vi "NumericArrayResizeTest.vi"() -> ()   [LabVIEW 2010]
uses:
  new_bsvt_test/Debug/new_bsvt_test.dll
panel:
  out "initialized array":i8[](array[numeric])
  out "size(s)":i32
  out "return type":i8
  out "arg1":i8[](array[numeric])
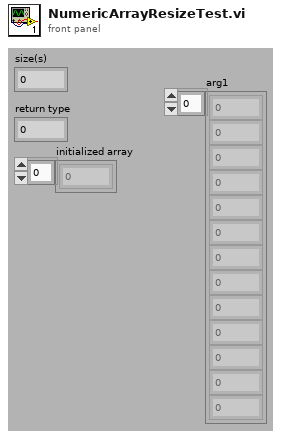
[diagram p1: front panel]
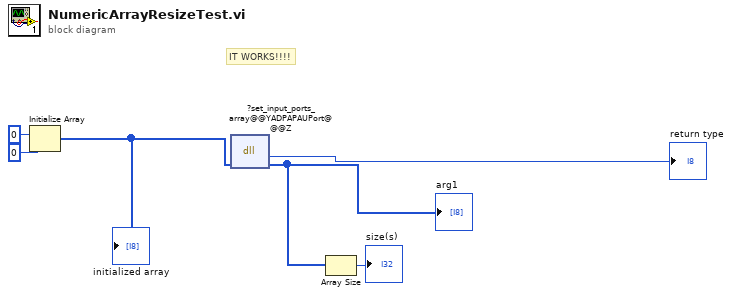
[diagram p0: block diagram]
diagram:
  # "IT WORKS!!!!"
  n1 = Initialize Array(i8 0 ("element"), 0 ("dimension size")) -> (w4:i8[])
  "initialized array" <- w4
  n2 = dll-call lib="D:/Liakh Tanya/Dissertation/Complex/DLL-s/new_bsvt_test/Debug/new_bsvt_test.dll" fn="?set_input_ports_array@@YADPAPAUPort@@@Z"("arg1"=w4) -> ("return type"=→"return type":i8, "arg1"=w2:i8[])  [unwired: 3 in, 2 out]
  "arg1" <- w2
  n3 = Array Size(array=w2) -> (size(s)=→"size(s)":i32)
